vi "NMRFMswitch.vi"() -> ()   [LabVIEW 2018]
uses:
  <vilib>/Analysis/2dsp.llb/Power Spectrum (DBL).vi
  rssmt/RunNumberGlobal.vi
  kleinjan/MKS/Global - Pressure & Flow.vi
  <vilib>/Analysis/NI_AALBase.lvlib
  <vilib>/Analysis/NI_AALPro.lvlib
panel:
  in  "RunNumber":dbl format="%#_13g"
  out "Peak Amp":dbl(graph)=74.1337708971354
  out "Python OK":bool=TRUE
  out "Polarization":sgl=1.7080129 format="%.3f"
  out "+3.3V OK":bool=TRUE
  out "Qsub OK":bool
  out "standard error":string
  out "standard output":string
  out "return code":i32
  out "initphase":dbl=2.09 format="%#_13g"
  out "inittune":dbl=3.248 format="%#_13g"
  in  "Save Tune":bool
  in  "Tune?":bool=TRUE
  out "Date / Time":string="12/21/2021 3:07:32 PM"
  in  "Stop Run":bool=TRUE
  out "He readback":bool
  in  "Prompt?":bool
  out "He temp (K)":sgl=2.13326 format="%.3f"
  out "He press (torr)":sgl=33.89 format="%.3f"
  in  "NMR Channel Select":string(combo)="Tune1.csv"
  out "Color Box":u32(colorbox)=16711680
  out "Measurement":enum16{"TEQ", "POL", "QCV"}(ring)=enum."QCV"
  in  "VME IP Address":string="192.168.24.146"
  out "FFT Vrms":dbl[](graph)=[0.005219076637020729, 0.0039878980940110925, 0.0036329447037529434, 0.003167506199185892, 0.002848999314516927, 0.0024923420584089507, 0.002185783432691833, 0.0019623062753076612, 0.0017456237192042675, 0.0015310589705579407, 0.0013569206947159228, 0.0012134296553531008, 0.0010661913882126185, 0.0009417865401198701, 0.0008289553058562431, 0.0007426697969914733, 0.0006543871227562969, 0.0005691981056566225, 0.0004985796296117873, 0.000444582165316538, 0.0003908334146047696, 0.00034689887876954856, 0.00029774652842368897, 0.0002704403862780026, 0.0002271604793132453, 0.00020413555661144572, 0.00017624411940442264, 0.00015585149747815723, 0.00013132078167075022, 0.0001195156866464364, 0.00010987586628788737, 8.462443756275535e-05, 7.876977088235619e-05, 6.70471531529734e-05, 6.782696234467443e-05, 5.204485709629659e-05, 4.2881690215771905e-05, 2.868837131108542e-05, 3.646022540118467e-05, 2.5174670763212626e-05, 2.4275865918577663e-05, 1.977860163321803e-05, 2.0218195658450144e-05, 1.5094086218758437e-05, 1.0805592250755934e-05, 1.1612054327236393e-05, 1.0702829004656882e-05, 6.927920054257791e-06, 8.444237907182155e-06, 4.302452084273682e-06, 5.339321799968253e-06, 7.218121245343906e-06, 3.7765728081436e-06, 2.8602044585862934e-06, 4.859347329579347e-06, 5.065161881862085e-06, 2.3556171895703534e-06, 1.7632661431426266e-06, 3.379390145710016e-06, 2.7603757096228226e-06, 3.6214619183540137e-06, 3.3344073928151306e-06, 1.102179735422125e-06, 1.0412493305540784e-05, 2.523883779132704e-06, 5.9409226720671005e-06, 3.4619760167465126e-07, 9.010440109742317e-07, 2.401774338798568e-07, 5.3535552158452226e-06, 3.6940163929523105e-06, 3.4039009222603295e-06, 4.582524510322615e-06, 2.513437155372671e-06, 3.895119393056086e-06, 7.346211597269102e-06, 7.126116644995652e-06, 6.049774016482352e-06, 8.854330148411976e-06, 9.192536011516818e-07, 7.232552250072598e-06, 7.328129506360153e-06, 6.413204468246682e-06, 6.579066941521174e-06, 4.988346286272407e-06, 3.865009185428311e-06, 5.9602567586528205e-06, 6.379649198485404e-06, 1.9180240572629512e-06, 2.4865392439123074e-06, 4.077423508916666e-06, 2.6143194254198198e-06, 1.1582615724765671e-06, 2.8823995318867116e-06, 6.385725297552865e-06, 7.387976979956906e-06, 1.962928382011928e-06, 5.487268486039249e-06, 4.542898540052593e-06, 3.920885322308244e-06, 2.560006411681713e-06, 6.030758252294827e-06, 2.8147731643947036e-06, 3.767037305710274e-06, 2.2940292462848864e-06, 6.082474368564689e-07, 3.32627146099113e-06, 1.4201614366018455e-06, 2.990764004313556e-06, 5.798579609053757e-06, 8.551040913858013e-06, 6.487437175474049e-06, 5.280254351335599e-06, 3.2689120370825972e-06, 3.024531763084045e-06, 5.816131915181896e-06, 2.084880682526168e-06, 4.749183768250868e-06, 2.5155270391606587e-06, 5.161404132650414e-06, 8.948372740255112e-06, 3.7134069338070665e-06, 1.0504243435692216e-06, 2.486546756935266e-06, 5.708480201850752e-06, 3.4078826415869943e-06, 2.7526388449297627e-06, 8.105361535117322e-06, 1.4868612920884835e-06, 2.3496303492346643e-06, 3.1063386478581925e-06, 1.6041115487796047e-06, 2.5868779778952035e-06, 5.345577459310027e-06, 1.9006938798563804e-06, 4.397705633197135e-06, 3.38743005875455e-06, 1.4982947809591981e-06, 2.6902031437364864e-06, 3.732947753472797e-06, 2.3609284770920314e-06, 9.243175552374334e-06, 3.912353690878166e-06, 4.4078681623996285e-06, 3.838535836859122e-06, 3.3526472596387042e-06, 4.571851526932495e-06, 2.4329647044319065e-06, 2.497090370438281e-06, 4.215928959236651e-06, 4.9956874449258715e-06, 3.993018282604913e-06, 4.835554673477225e-06, 2.6850490929158865e-06, 4.737311136731914e-06, 1.9370086076116144e-06, 1.6342895919624075e-06, 1.5865940297551477e-06, 2.3464563158779775e-06, 3.8000988173413713e-06, 2.3042989349919555e-06, 4.252040733881927e-06, 5.922353590007147e-06, 4.960033169847504e-06, 8.415695746076422e-07, 2.5973560267739965e-06, 4.145285922687817e-06, 1.4972808238134822e-06, 3.6651950916562555e-06, 7.692102378806355e-06, 2.252172769669826e-06, 2.528448476027188e-06, 1.7270842871089151e-06, 8.732998643384956e-07, 1.941128023169817e-06, 4.967581144990737e-07, 2.122261572666148e-06, 2.7403051949501256e-06, 2.4487149582217077e-06, 4.695501688085451e-06, 4.028757067113805e-06, 3.994650398277535e-06, 1.321960383008639e-06, 7.229471979478003e-06, 2.8630109874025474e-06, 4.835926382490523e-06, 5.328936669165124e-06, 3.2295568028357553e-06, 4.122039456315995e-06, 4.415345749314911e-06, 2.0464868375281003e-06, 2.116876710242299e-06, 4.34647621603492e-06, 7.346635334484221e-06, 3.735213245442724e-06, 1.4876587271631782e-06, 2.3704959917761274e-06, 2.23938979663892e-06, 3.6731417379864763e-06, 2.541846286331768e-06, 1.6299280662148296e-06, 1.6299280662148296e-06, 2.541846286331768e-06, 3.6731417379864763e-06, 2.23938979663892e-06, 2.3704959917761274e-06, 1.4876587271631782e-06, 3.735213245442724e-06, 7.346635334484221e-06, 4.34647621603492e-06, 2.116876710242299e-06, 2.0464868375281003e-06, 4.415345749314911e-06, 4.122039456315995e-06, 3.2295568028357553e-06, 5.328936669165124e-06, 4.835926382490523e-06, 2.8630109874025474e-06, 7.229471979478003e-06, 1.321960383008639e-06, 3.994650398277535e-06, 4.028757067113805e-06, 4.695501688085451e-06, 2.4487149582217077e-06, 2.7403051949501256e-06, 2.122261572666148e-06, 4.967581144990737e-07, 1.941128023169817e-06, 8.732998643384956e-07, 1.7270842871089151e-06, 2.528448476027188e-06, 2.252172769669826e-06, 7.692102378806355e-06, 3.6651950916562555e-06, 1.4972808238134822e-06, 4.145285922687817e-06, 2.5973560267739965e-06, 8.415695746076422e-07, 4.960033169847504e-06, 5.922353590007147e-06, 4.252040733881927e-06, 2.3042989349919555e-06, 3.8000988173413713e-06, 2.3464563158779775e-06, 1.5865940297551477e-06, 1.6342895919624075e-06, 1.9370086076116144e-06, 4.737311136731914e-06, 2.6850490929158865e-06, 4.835554673477225e-06, 3.993018282604913e-06, 4.9956874449258715e-06, 4.215928959236651e-06, 2.497090370438281e-06, 2.4329647044319065e-06, 4.571851526932495e-06, 3.3526472596387042e-06, 3.838535836859122e-06, 4.4078681623996285e-06, 3.912353690878166e-06, 9.243175552374334e-06, 2.3609284770920314e-06, 3.732947753472797e-06, 2.6902031437364864e-06, 1.4982947809591981e-06, 3.38743005875455e-06, 4.397705633197135e-06, 1.9006938798563804e-06, 5.345577459310027e-06, 2.5868779778952035e-06, 1.6041115487796047e-06, 3.1063386478581925e-06, 2.3496303492346643e-06, 1.4868612920884835e-06, 8.105361535117322e-06, 2.7526388449297627e-06, 3.4078826415869943e-06, 5.708480201850752e-06, 2.486546756935266e-06, 1.0504243435692216e-06, 3.7134069338070665e-06, 8.948372740255112e-06, 5.161404132650414e-06, 2.5155270391606587e-06, 4.749183768250868e-06, 2.084880682526168e-06, 5.816131915181896e-06, 3.024531763084045e-06, 3.2689120370825972e-06, 5.280254351335599e-06, 6.487437175474049e-06, 8.551040913858013e-06, 5.798579609053757e-06, 2.990764004313556e-06, 1.4201614366018455e-06, 3.32627146099113e-06, 6.082474368564689e-07, 2.2940292462848864e-06, 3.767037305710274e-06, 2.8147731643947036e-06, 6.030758252294827e-06, 2.560006411681713e-06, 3.920885322308244e-06, 4.542898540052593e-06, 5.487268486039249e-06, 1.962928382011928e-06, 7.387976979956906e-06, 6.385725297552865e-06, 2.8823995318867116e-06, 1.1582615724765671e-06, 2.6143194254198198e-06, 4.077423508916666e-06, 2.4865392439123074e-06, 1.9180240572629512e-06, 6.379649198485404e-06, 5.9602567586528205e-06, 3.865009185428311e-06, 4.988346286272407e-06, 6.579066941521174e-06, 6.413204468246682e-06, 7.328129506360153e-06, 7.232552250072598e-06, 9.192536011516818e-07, 8.854330148411976e-06, 6.049774016482352e-06, 7.126116644995652e-06, 7.346211597269102e-06, 3.895119393056086e-06, 2.513437155372671e-06, 4.582524510322615e-06, 3.4039009222603295e-06, 3.6940163929523105e-06, 5.3535552158452226e-06, 2.401774338798568e-07, 9.010440109742317e-07, 3.4619760167465126e-07, 5.9409226720671005e-06, 2.523883779132704e-06, 1.0412493305540784e-05, 1.102179735422125e-06, 3.3344073928151306e-06, 3.6214619183540137e-06, 2.7603757096228226e-06, 3.379390145710016e-06, 1.7632661431426266e-06, 2.3556171895703534e-06, 5.065161881862085e-06, 4.859347329579347e-06, 2.8602044585862934e-06, 3.7765728081436e-06, 7.218121245343906e-06, 5.339321799968253e-06, 4.302452084273682e-06, 8.444237907182155e-06, 6.927920054257791e-06, 1.0702829004656882e-05, 1.1612054327236393e-05, 1.0805592250755934e-05, 1.5094086218758437e-05, 2.0218195658450144e-05, 1.977860163321803e-05, 2.4275865918577663e-05, 2.5174670763212626e-05, 3.646022540118467e-05, 2.868837131108542e-05, 4.2881690215771905e-05, 5.204485709629659e-05, 6.782696234467443e-05, 6.70471531529734e-05, 7.876977088235619e-05, 8.462443756275535e-05, 0.00010987586628788737, 0.0001195156866464364, 0.00013132078167075022, 0.00015585149747815723, 0.00017624411940442264, 0.00020413555661144572, 0.0002271604793132453, 0.0002704403862780026, 0.00029774652842368897, 0.00034689887876954856, 0.0003908334146047696, 0.000444582165316538, 0.0004985796296117873, 0.0005691981056566225, 0.0006543871227562969, 0.0007426697969914733, 0.0008289553058562431, 0.0009417865401198701, 0.0010661913882126185, 0.0012134296553531008, 0.0013569206947159228, 0.0015310589705579407, 0.0017456237192042675, 0.0019623062753076612, 0.002185783432691833, 0.0024923420584089507, 0.002848999314516927, 0.003167506199185892, 0.0036329447037529434, 0.0039878980940110925]
  out "Raw NMR Graph / Ave":cluster{dbl, "Step Width (MHz)":dbl, dbl[][]}(graph)={224.25, "Step Width (MHz)"=0.001, [[0.0013885498046875, 0.001312255859375, 0.0015411376953125, 0.0014190673828125, 0.00146484375, 0.0015106201171875, 0.00146484375, 0.0014801025390625, 0.001434326171875, 0.001373291015625, 0.0012969970703125, 0.0012969970703125, 0.0012969970703125, 0.00140380859375, 0.001373291015625, 0.0013275146484375, 0.001373291015625, 0.0013885498046875, 0.001373291015625, 0.0013427734375, 0.0013580322265625, 0.001495361328125, 0.0012969970703125, 0.0011138916015625, 0.0013885498046875, 0.001251220703125, 0.0012969970703125, 0.001220703125, 0.001220703125, 0.0013275146484375, 0.00140380859375, 0.00140380859375, 0.00146484375, 0.0013427734375, 0.0012359619140625, 0.00140380859375, 0.0012664794921875, 0.001312255859375, 0.0013427734375, 0.00128173828125, 0.001129150390625, 0.0012359619140625, 0.0012664794921875, 0.0012054443359375, 0.0012054443359375, 0.0012664794921875, 0.0012359619140625, 0.001220703125, 0.001129150390625, 0.000946044921875, 0.0012359619140625, 0.0010833740234375, 0.0010986328125, 0.001068115234375, 0.0012054443359375, 0.00115966796875, 0.0012359619140625, 0.00115966796875, 0.0010223388671875, 0.001068115234375, 0.001220703125, 0.0011138916015625, 0.00103759765625, 0.0010833740234375, 0.0010528564453125, 0.0009307861328125, 0.000946044921875, 0.001068115234375, 0.001190185546875, 0.00115966796875, 0.001190185546875, 0.0012969970703125, 0.0012664794921875, 0.0010528564453125, 0.001129150390625, 0.001312255859375, 0.001190185546875, 0.0011138916015625, 0.001129150390625, 0.0011444091796875, 0.0011749267578125, 0.0012359619140625, 0.0010833740234375, 0.001190185546875, 0.0010833740234375, 0.0011444091796875, 0.001129150390625, 0.001190185546875, 0.0013580322265625, 0.0013275146484375, 0.0012969970703125, 0.00128173828125, 0.001251220703125, 0.00115966796875, 0.001220703125, 0.0013580322265625, 0.0012969970703125, 0.0012664794921875, 0.0013885498046875, 0.0013580322265625, 0.001434326171875, 0.0015106201171875, 0.0014190673828125, 0.001312255859375, 0.0015411376953125, 0.0013580322265625, 0.001190185546875, 0.001556396484375, 0.001495361328125, 0.001495361328125, 0.0015869140625, 0.0015869140625, 0.00152587890625, 0.0016937255859375, 0.001708984375, 0.0017852783203125, 0.001556396484375, 0.00152587890625, 0.0017852783203125, 0.0016326904296875, 0.0016937255859375, 0.00177001953125, 0.00177001953125, 0.0018463134765625, 0.00189208984375, 0.0018463134765625, 0.0019073486328125, 0.0017852783203125, 0.0019378662109375, 0.001922607421875, 0.002044677734375, 0.00201416015625, 0.001983642578125, 0.002044677734375, 0.0020751953125, 0.0022735595703125, 0.002227783203125, 0.0022430419921875, 0.0023345947265625, 0.00244140625, 0.002471923828125, 0.0027008056640625, 0.0025787353515625, 0.002685546875, 0.0028228759765625, 0.0028839111328125, 0.0029296875, 0.003143310546875, 0.003143310546875, 0.0031585693359375, 0.0032501220703125, 0.0034637451171875, 0.003570556640625, 0.0037078857421875, 0.00390625, 0.0040740966796875, 0.0041351318359375, 0.0042572021484375, 0.0045013427734375, 0.0045623779296875, 0.0048675537109375, 0.0052032470703125, 0.00543212890625, 0.005645751953125, 0.0059967041015625, 0.006378173828125, 0.00665283203125, 0.0069732666015625, 0.00738525390625, 0.007904052734375, 0.0084228515625, 0.0091400146484375, 0.009552001953125, 0.0103302001953125, 0.0110015869140625, 0.0119171142578125, 0.0129852294921875, 0.0140533447265625, 0.0154876708984375, 0.016815185546875, 0.0185546875, 0.02069091796875, 0.0230865478515625, 0.0256195068359375, 0.02874755859375, 0.0323333740234375, 0.0367584228515625, 0.0414581298828125, 0.046661376953125, 0.0526123046875, 0.058868408203125, 0.0647125244140625, 0.06964111328125, 0.0731658935546875, 0.074798583984375, 0.0745697021484375, 0.0721588134765625, 0.0679473876953125, 0.062469482421875, 0.05633544921875, 0.0499114990234375, 0.044036865234375, 0.0384979248046875, 0.033599853515625, 0.0293121337890625, 0.025787353515625, 0.02276611328125, 0.0201416015625, 0.017913818359375, 0.0159759521484375, 0.0142974853515625, 0.0130767822265625, 0.0119171142578125, 0.0106658935546875, 0.0097808837890625, 0.00909423828125, 0.00830078125, 0.00762939453125, 0.00714111328125, 0.0065765380859375, 0.006256103515625, 0.0059051513671875, 0.005462646484375, 0.005126953125, 0.004852294921875, 0.0044097900390625, 0.0040435791015625, 0.0039520263671875, 0.004150390625, 0.0038604736328125, 0.0036163330078125, 0.0033416748046875, 0.0032806396484375, 0.0029449462890625, 0.0030975341796875, 0.002716064453125, 0.002532958984375, 0.00244140625, 0.002532958984375, 0.0022430419921875, 0.002349853515625, 0.0022430419921875, 0.00213623046875, 0.0021514892578125, 0.0018463134765625, 0.001983642578125, 0.0017852783203125, 0.00177001953125, 0.0017852783203125, 0.0018157958984375, 0.0015869140625, 0.00164794921875, 0.001617431640625, 0.0017242431640625, 0.0016021728515625, 0.0014495849609375, 0.0013427734375, 0.0012969970703125, 0.00140380859375, 0.0011749267578125, 0.0012969970703125, 0.0012359619140625, 0.0011138916015625, 0.001190185546875, 0.0011138916015625, 0.0013427734375, 0.001190185546875, 0.00115966796875, 0.0010986328125, 0.0010833740234375, 0.001068115234375, 0.0010833740234375, 0.00115966796875, 0.0010528564453125, 0.001190185546875, 0.0011749267578125, 0.001068115234375, 0.000946044921875, 0.0009613037109375, 0.0009765625, 0.0012054443359375, 0.000885009765625, 0.0010986328125, 0.0009613037109375, 0.0008697509765625, 0.001068115234375, 0.0010223388671875, 0.001129150390625, 0.0010528564453125, 0.0012359619140625, 0.0012359619140625, 0.001129150390625, 0.0012664794921875, 0.00115966796875, 0.0012664794921875, 0.001068115234375, 0.0012054443359375, 0.0014190673828125, 0.001434326171875, 0.001312255859375, 0.001312255859375, 0.00115966796875, 0.0012359619140625, 0.0013580322265625, 0.00115966796875, 0.001190185546875, 0.0010223388671875, 0.000946044921875, 0.00103759765625, 0.0010833740234375, 0.0008392333984375, 0.0009307861328125, 0.0008392333984375, 0.0009765625, 0.000823974609375, 0.0008087158203125, 0.0007171630859375, 0.0007781982421875, 0.0007476806640625, 0.0008544921875, 0.0006256103515625, 0.0007476806640625, 0.00091552734375, 0.000762939453125, 0.0006866455078125, 0.0008544921875, 0.00067138671875, 0.0007476806640625, 0.000732421875, 0.00067138671875, 0.000762939453125, 0.0007476806640625, 0.0008087158203125, 0.0006866455078125, 0.000640869140625, 0.0005950927734375, 0.000640869140625, 0.000946044921875, 0.00067138671875, 0.0007476806640625, 0.00079345703125, 0.0009002685546875, 0.0008544921875, 0.00067138671875, 0.00079345703125, 0.0008087158203125, 0.000885009765625, 0.000823974609375, 0.0007476806640625, 0.0008087158203125, 0.0008697509765625, 0.000823974609375, 0.0008392333984375, 0.0009307861328125, 0.0007781982421875, 0.000732421875, 0.000762939453125, 0.0008697509765625, 0.0006866455078125, 0.0006256103515625, 0.000823974609375, 0.0009307861328125, 0.0008392333984375, 0.001068115234375, 0.0008087158203125, 0.0008087158203125, 0.0009307861328125, 0.001068115234375, 0.000946044921875, 0.0009002685546875, 0.0008697509765625, 0.001129150390625, 0.0010986328125, 0.00091552734375, 0.001068115234375, 0.0009002685546875, 0.00091552734375, 0.0009765625, 0.0009613037109375, 0.000823974609375, 0.0008087158203125, 0.00103759765625, 0.0012969970703125, 0.0009918212890625, 0.00103759765625, 0.0010528564453125, 0.0011138916015625, 0.000946044921875, 0.0010528564453125, 0.0010528564453125, 0.00091552734375, 0.0010833740234375, 0.0010986328125, 0.00115966796875, 0.001190185546875, 0.001220703125, 0.001251220703125, 0.0011138916015625, 0.0012359619140625, 0.0012359619140625, 0.001312255859375], [0.0, 0.0, 0.0, 0.0, 0.0, 0.0, 0.0, 0.0, 0.0, 0.0, 0.0, 0.0, 0.0, 0.0, 0.0, 0.0, 0.0, 0.0, 0.0, 0.0, 0.0, 0.0, 0.0, 0.0, 0.0, 0.0, 0.0, 0.0, 0.0, 0.0, 0.0, 0.0, 0.0, 0.0, 0.0, 0.0, 0.0, 0.0, 0.0, 0.0, 0.0, 0.0, 0.0, 0.0, 0.0, 0.0, 0.0, 0.0, 0.0, 0.0, 0.0, 0.0, 0.0, 0.0, 0.0, 0.0, 0.0, 0.0, 0.0, 0.0, 0.0, 0.0, 0.0, 0.0, 0.0, 0.0, 0.0, 0.0, 0.0, 0.0, 0.0, 0.0, 0.0, 0.0, 0.0, 0.0, 0.0, 0.0, 0.0, 0.0, 0.0, 0.0, 0.0, 0.0, 0.0, 0.0, 0.0, 0.0, 0.0, 0.0, 0.0, 0.0, 0.0, 0.0, 0.0, 0.0, 0.0, 0.0, 0.0, 0.0, 0.0, 0.0, 0.0, 0.0, 0.0, 0.0, 0.0, 0.0, 0.0, 0.0, 0.0, 0.0, 0.0, 0.0, 0.0, 0.0, 0.0, 0.0, 0.0, 0.0, 0.0, 0.0, 0.0, 0.0, 0.0, 0.0, 0.0, 0.0, 0.0, 0.0, 0.0, 0.0, 0.0, 0.0, 0.0, 0.0, 0.0, 0.0, 0.0, 0.0, 0.0, 0.0, 0.0, 0.0, 0.0, 0.0, 0.0, 0.0, 0.0, 0.0, 0.0, 0.0, 0.0, 0.0, 0.0, 0.0, 0.0, 0.0, 0.0, 0.0, 0.0, 0.0, 0.0, 0.0, 0.0, 0.0, 0.0, 0.0, 0.0, 0.0, 0.0, 0.0, 0.0, 0.0, 0.0, 0.0, 0.0, 0.0, 0.0, 0.0, 0.0, 0.0, 0.0, 0.0, 0.0, 0.0, 0.0, 0.0, 0.0, 0.0, 0.0, 0.0, 0.0, 0.0, 0.0, 0.0, 0.0, 0.0, 0.0, 0.0, 0.0, 0.0, 0.0, 0.0, 0.0, 0.0, 0.0, 0.0, 0.0, 0.0, 0.0, 0.0, 0.0, 0.0, 0.0, 0.0, 0.0, 0.0, 0.0, 0.0, 0.0, 0.0, 0.0, 0.0, 0.0, 0.0, 0.0, 0.0, 0.0, 0.0, 0.0, 0.0, 0.0, 0.0, 0.0, 0.0, 0.0, 0.0, 0.0, 0.0, 0.0, 0.0, 0.0, 0.0, 0.0, 0.0, 0.0, 0.0, 0.0, 0.0, 0.0, 0.0, 0.0, 0.0, 0.0, 0.0, 0.0, 0.0, 0.0, 0.0, 0.0, 0.0, 0.0, 0.0, 0.0, 0.0, 0.0, 0.0, 0.0, 0.0, 0.0, 0.0, 0.0, 0.0, 0.0, 0.0, 0.0, 0.0, 0.0, 0.0, 0.0, 0.0, 0.0, 0.0, 0.0, 0.0, 0.0, 0.0, 0.0, 0.0, 0.0, 0.0, 0.0, 0.0, 0.0, 0.0, 0.0, 0.0, 0.0, 0.0, 0.0, 0.0, 0.0, 0.0, 0.0, 0.0, 0.0, 0.0, 0.0, 0.0, 0.0, 0.0, 0.0, 0.0, 0.0, 0.0, 0.0, 0.0, 0.0, 0.0, 0.0, 0.0, 0.0, 0.0, 0.0, 0.0, 0.0, 0.0, 0.0, 0.0, 0.0, 0.0, 0.0, 0.0, 0.0, 0.0, 0.0, 0.0, 0.0, 0.0, 0.0, 0.0, 0.0, 0.0, 0.0, 0.0, 0.0, 0.0, 0.0, 0.0, 0.0, 0.0, 0.0, 0.0, 0.0, 0.0, 0.0, 0.0, 0.0, 0.0, 0.0, 0.0, 0.0, 0.0, 0.0, 0.0, 0.0, 0.0, 0.0, 0.0, 0.0, 0.0, 0.0, 0.0, 0.0, 0.0, 0.0, 0.0, 0.0, 0.0, 0.0, 0.0, 0.0, 0.0, 0.0, 0.0, 0.0, 0.0, 0.0, 0.0, 0.0, 0.0, 0.0, 0.0, 0.0, 0.0, 0.0, 0.0, 0.0, 0.0, 0.0], [0.000884405500000046, 0.000875605500000004, 0.0008668494999999623, 0.0008581375000001678, 0.0008494695000001258, 0.000840845500000084, 0.0008322655000000428, 0.0008237295000000018, 0.0008152374999999615, 0.0008067895000001609, 0.00079838550000012, 0.0007900255000000796, 0.0007817095000000395, 0.0007734374999999999, 0.0007652094999999607, 0.0007570255000001541, 0.0007488855000001145, 0.0007407895000000752, 0.0007327375000000365, 0.0007247294999999981, 0.0007167654999999602, 0.0007088455000001472, 0.0007009695000001089, 0.0006931375000000709, 0.0006853495000000335, 0.0006776054999999964, 0.0006699054999999598, 0.0006622495000001405, 0.0006546375000001035, 0.0006470695000000669, 0.0006395455000000307, 0.0006320654999999949, 0.0006246294999999595, 0.000617237500000134, 0.0006098895000000983, 0.0006025855000000629, 0.0005953255000000279, 0.0005881094999999934, 0.0005809374999999593, 0.0005738095000001277, 0.0005667255000000931, 0.000559685500000059, 0.0005526895000000253, 0.0005457374999999921, 0.0005388294999999593, 0.0005319655000001213, 0.0005251455000000881, 0.0005183695000000552, 0.0005116375000000228, 0.0005049494999999909, 0.0004983054999999593, 0.0004917055000001151, 0.00048514950000008315, 0.0004786375000000516, 0.0004721695000000205, 0.00046574549999998976, 0.0004593654999999595, 0.0004530295000001091, 0.0004467375000000784, 0.0004404895000000481, 0.00043428550000001824, 0.0004281254999999888, 0.0004220094999999598, 0.0004159375000001032, 0.0004099095000000737, 0.00040392550000004475, 0.0003979855000000161, 0.00039208949999998795, 0.0003862374999999602, 0.0003804295000000973, 0.0003746655000000691, 0.00036894550000004145, 0.00036326950000001415, 0.0003576374999999872, 0.0003520494999999607, 0.00034650550000009167, 0.00034100550000006475, 0.0003355495000000383, 0.00033013750000001225, 0.0003247694999999866, 0.0003194454999999614, 0.0003141655000000861, 0.00030892950000006045, 0.00030373750000003524, 0.00029858950000001045, 0.00029348549999998614, 0.00028842549999996215, 0.0002834095000000806, 0.00027843750000005626, 0.00027350950000003233, 0.00026862550000000883, 0.00026378549999998575, 0.0002589894999999631, 0.00025423750000007524, 0.0002495295000000522, 0.00024486550000002953, 0.00024024550000000731, 0.00023566949999998546, 0.00023113749999996411, 0.00022664950000007007, 0.00022220550000004826, 0.00021780550000002687, 0.00021344950000000589, 0.00020913749999998534, 0.00020486949999996525, 0.00020064550000006495, 0.00019646550000004443, 0.0001923295000000243, 0.0001882375000000046, 0.00018418949999998537, 0.00018018549999996648, 0.00017622550000005998, 0.0001723095000000407, 0.00016843750000002187, 0.00016460950000000345, 0.00016082549999998544, 0.00015708549999996787, 0.00015338950000005512, 0.00014973750000003713, 0.00014612950000001957, 0.0001425655000000024, 0.00013904549999998566, 0.00013556949999996937, 0.0001321375000000504, 0.00012874950000003367, 0.00012540550000001736, 0.00012210550000000148, 0.00011884949999998602, 0.00011563750000006164, 0.00011246950000004579, 0.00010934550000003033, 0.00010626550000001528, 0.00010322950000000068, 0.00010023749999998649, 9.728950000005588e-05, 9.438550000004129e-05, 9.152550000002709e-05, 8.870950000001334e-05, 8.59375e-05, 8.320949999998707e-05, 8.052550000005024e-05, 7.78855000000369e-05, 7.528950000002399e-05, 7.273750000001149e-05, 7.022949999999943e-05, 6.776549999998778e-05, 6.534550000004471e-05, 6.296950000003266e-05, 6.0637500000021e-05, 5.8349500000009786e-05, 5.6105499999998984e-05, 5.390549999998861e-05, 5.17495000000393e-05, 4.963750000002851e-05, 4.756950000001814e-05, 4.554550000000819e-05, 4.356549999999866e-05, 4.162949999998955e-05, 3.9737500000034014e-05, 3.788950000002449e-05, 3.6085500000015394e-05, 3.432550000000672e-05, 3.260949999999846e-05, 3.093749999999062e-05, 2.9309500000028848e-05, 2.77255000000206e-05, 2.618550000001277e-05, 2.468950000000536e-05, 2.3237499999998376e-05, 2.1829499999991806e-05, 2.0465500000023797e-05, 1.914550000001682e-05, 1.7869500000010265e-05, 1.6637500000004125e-05, 1.5449499999998406e-05, 1.430549999999311e-05, 1.3205500000018873e-05, 1.2149500000013166e-05, 1.1137500000007877e-05, 1.016950000000301e-05, 9.245499999998563e-06, 8.365499999994538e-06, 7.5295000000140655e-06, 6.7375000000096285e-06, 5.989500000005612e-06, 5.2855000000020156e-06, 4.625499999998839e-06, 4.009499999996083e-06, 3.4375000000093793e-06, 2.9095000000062124e-06, 2.4255000000034664e-06, 1.9855000000011404e-06, 1.5894999999992347e-06, 1.237499999997749e-06, 9.295000000048122e-07, 6.655000000029163e-07, 4.455000000014406e-07, 2.6950000000038516e-07, 1.374999999997499e-07, 4.9499999999534794e-08, 5.500000000365162e-09, 5.499999999739884e-09, 4.9499999999534794e-08, 1.374999999997499e-07, 2.6950000000038516e-07, 4.455000000014406e-07, 6.654999999960382e-07, 9.294999999966835e-07, 1.237499999997749e-06, 1.5894999999992347e-06, 1.9855000000011404e-06, 2.4255000000034664e-06, 2.9094999999918315e-06, 3.437499999993747e-06, 4.009499999996083e-06, 4.625499999998839e-06, 5.2855000000020156e-06, 5.989500000005612e-06, 6.737499999987744e-06, 7.5294999999909305e-06, 8.365499999994538e-06, 9.245499999998563e-06, 1.016950000000301e-05, 1.1137500000007877e-05, 1.2149499999983777e-05, 1.3205499999988236e-05, 1.430549999999311e-05, 1.5449499999998406e-05, 1.6637500000004125e-05, 1.7869500000010265e-05, 1.914549999997993e-05, 2.0465499999985657e-05, 2.1829499999991806e-05, 2.3237499999998376e-05, 2.468950000000536e-05, 2.618550000001277e-05, 2.7725499999976206e-05, 2.93094999999832e-05, 3.093749999999062e-05, 3.260949999999846e-05, 3.432550000000672e-05, 3.6085500000015394e-05, 3.7889499999972594e-05, 3.973749999998087e-05, 4.162949999998955e-05, 4.356549999999866e-05, 4.554550000000819e-05, 4.756950000001814e-05, 4.9637499999969114e-05, 5.174949999997865e-05, 5.390549999998861e-05, 5.6105499999998984e-05, 5.8349500000009786e-05, 6.0637499999955355e-05, 6.296949999996573e-05, 6.534549999997655e-05, 6.776549999998778e-05, 7.022949999999943e-05, 7.273750000001149e-05, 7.528949999995083e-05, 7.788549999996248e-05, 8.052549999997458e-05, 8.320949999998707e-05, 8.59375e-05, 8.870950000001334e-05, 9.152549999994642e-05, 9.438549999995936e-05, 9.728949999997272e-05, 0.00010023749999998649, 0.00010322950000000068, 0.00010626550000001528, 0.00010934549999994216, 0.00011246949999995637, 0.00011563749999997098, 0.00011884949999998602, 0.00012210550000000148, 0.00012540550000001736, 0.000128749499999938, 0.00013213749999995347, 0.00013556949999996937, 0.00013904549999998566, 0.0001425655000000024, 0.00014612950000001957, 0.00014973749999993397, 0.0001533894999999507, 0.00015708549999996787, 0.00016082549999998544, 0.00016460950000000345, 0.00016843750000002187, 0.00017230949999993004, 0.00017622549999994806, 0.00018018549999996648, 0.00018418949999998537, 0.0001882375000000046, 0.0001923295000000243, 0.00019646549999992622, 0.00020064549999994553, 0.00020486949999996525, 0.00020913749999998534, 0.00021344950000000589, 0.00021780550000002687, 0.00022220549999992255, 0.00022664949999994313, 0.00023113749999996411, 0.00023566949999998546, 0.00024024550000000731, 0.00024486550000002953, 0.000249529499999919, 0.00025423749999994085, 0.0002589894999999631, 0.00026378549999998575, 0.00026862550000000883, 0.00027350950000003233, 0.0002784374999999156, 0.0002834094999999387, 0.00028842549999996215, 0.00029348549999998614, 0.00029858950000001045, 0.00030373750000003524, 0.00030892949999991224, 0.0003141654999999366, 0.0003194454999999614, 0.0003247694999999866, 0.00033013750000001225, 0.0003355495000000383, 0.00034100549999990906, 0.00034650549999993473, 0.0003520494999999607, 0.0003576374999999872, 0.00036326950000001415, 0.00036894550000004145, 0.00037466549999990594, 0.00038042949999993284, 0.0003862374999999602, 0.00039208949999998795, 0.0003979855000000161, 0.00040392550000004475, 0.00040990949999990305, 0.0004159374999999312, 0.0004220094999999598, 0.0004281254999999888, 0.00043428550000001824, 0.0004404895000000481, 0.00044673749999990016, 0.00045302949999992967, 0.0004593654999999595, 0.00046574549999998976, 0.0004721695000000205, 0.0004786375000000516, 0.00048514949999989743, 0.0004917054999999282, 0.0004983054999999593, 0.0005049494999999909, 0.0005116375000000228, 0.0005183695000000552, 0.0005251454999998949, 0.0005319654999999269, 0.0005388294999999593, 0.0005457374999999921, 0.0005526895000000253, 0.000559685500000059, 0.0005667254999998924, 0.0005738094999999257, 0.0005809374999999593, 0.0005881094999999934, 0.0005953255000000279, 0.0006025855000000629, 0.0006098894999998901, 0.0006172374999999246, 0.0006246294999999595, 0.0006320654999999949, 0.0006395455000000307, 0.0006470695000000669, 0.0006546374999998878, 0.0006622494999999236, 0.0006699054999999598, 0.0006776054999999964, 0.0006853495000000335, 0.000693137499999849, 0.0007009694999998856, 0.0007088454999999227, 0.0007167654999999602, 0.0007247294999999981, 0.0007327375000000365, 0.0007407894999998458, 0.0007488854999998836, 0.000757025499999922, 0.0007652094999999607, 0.0007734374999999999, 0.0007817095000000395, 0.0007900254999998427, 0.0007983854999998819, 0.0008067894999999214, 0.0008152374999999615, 0.0008237295000000018, 0.0008322655000000428, 0.0008408454999998396, 0.00084946949999988, 0.0008581374999999208, 0.0008668494999999623, 0.000875605500000004]]}
  in  "R&S GPIB Addr (28)":refnum<visa-resource-name>="GPIB0::28::INSTR"
  out "Pedestal (V)":dbl=0.0006638835872395818 format="%_2g"
  in  "Open Global Panel":bool=TRUE
  out "Peak center (MHz)":sgl=224.44414 format="%.3f"
  out "Telnet error out":errorcluster
  out "+3.3V supply":dbl=3.284 format="%_4g"
  out "Temp (C)":dbl=31.12 format="%_4g"
  out "RF level OK":bool=TRUE
  out "Polarization %":sgl=1.7080129 format="%.3e"
  out "# Good Spectra":i32=500
  out "Pedestal volts OK":bool=TRUE
  out "Sweep #":i32=6
  out "1st Sweep":bool
  out "ADC volts OK":bool=TRUE
  out "Peak Height Distribution":cluster{"Y":dbl[], "Y":dbl[]}[](graph)=[{"Y"=[1.68515093263186, 1.685512718520532, 1.6858745044092038, 1.6862362902978758, 1.6865980761865478, 1.6869598620752195, 1.6873216479638915, 1.6876834338525633, 1.6880452197412352, 1.688407005629907, 1.688768791518579, 1.6891305774072507, 1.6894923632959227, 1.6898541491845946, 1.6902159350732664, 1.6905777209619384, 1.6909395068506101, 1.691301292739282, 1.6916630786279538, 1.6920248645166258, 1.6923866504052976, 1.6927484362939695, 1.6931102221826415, 1.6934720080713133, 1.6938337939599852, 1.694195579848657, 1.694557365737329, 1.6949191516260007, 1.6952809375146727, 1.6956427234033447, 1.6960045092920164, 1.6963662951806884, 1.6967280810693601, 1.697089866958032, 1.6974516528467039, 1.6978134387353758, 1.6981752246240476, 1.6985370105127195, 1.6988987964013915, 1.6992605822900633, 1.6996223681787352, 1.699984154067407, 1.700345939956079, 1.7007077258447507, 1.7010695117334227, 1.7014312976220944, 1.7017930835107664, 1.7021548693994384, 1.7025166552881101, 1.702878441176782, 1.7032402270654539, 1.7036020129541258, 1.7039637988427976, 1.7043255847314696, 1.7046873706201415, 1.7050491565088133, 1.7054109423974853, 1.705772728286157, 1.706134514174829, 1.7064963000635007, 1.7068580859521727, 1.7072198718408444, 1.7075816577295164, 1.7079434436181884, 1.7083052295068601, 1.7086670153955321, 1.7090288012842039, 1.7093905871728758, 1.7097523730615476, 1.7101141589502196, 1.7104759448388913, 1.7108377307275633, 1.7111995166162353, 1.711561302504907, 1.711923088393579, 1.7122848742822507, 1.7126466601709227, 1.7130084460595945, 1.7133702319482664, 1.7137320178369384, 1.7140938037256102, 1.7144555896142821, 1.7148173755029539, 1.7151791613916259, 1.7155409472802976, 1.7159027331689696, 1.7162645190576413, 1.7166263049463133, 1.7169880908349853, 1.717349876723657, 1.717711662612329, 1.7180734485010007, 1.7184352343896727, 1.7187970202783445, 1.7191588061670164, 1.7195205920556882, 1.7198823779443602, 1.7202441638330321, 1.7206059497217039, 1.7209677356103759], "Y"=[1.0, 0.0, 1.0, 0.0, 2.0, 2.0, 2.0, 2.0, 0.0, 1.0, 1.0, 2.0, 2.0, 1.0, 0.0, 1.0, 1.0, 5.0, 0.0, 2.0, 1.0, 3.0, 1.0, 4.0, 3.0, 6.0, 3.0, 5.0, 2.0, 6.0, 8.0, 7.0, 8.0, 12.0, 12.0, 10.0, 9.0, 15.0, 3.0, 8.0, 11.0, 11.0, 9.0, 14.0, 14.0, 17.0, 9.0, 15.0, 13.0, 15.0, 9.0, 11.0, 9.0, 16.0, 7.0, 11.0, 9.0, 6.0, 8.0, 9.0, 8.0, 14.0, 8.0, 6.0, 8.0, 5.0, 6.0, 4.0, 5.0, 11.0, 4.0, 4.0, 1.0, 3.0, 5.0, 5.0, 5.0, 4.0, 2.0, 5.0, 1.0, 0.0, 1.0, 4.0, 1.0, 1.0, 1.0, 0.0, 0.0, 0.0, 1.0, 0.0, 0.0, 0.0, 0.0, 0.0, 1.0, 0.0, 0.0, 1.0]}]
  out "S/N":dbl=276.4068357498407 format="%_3g"
  out "Polarization %":dbl=1.7024247821191647 format="%_4g"
  out "Pedestal Diff (V)":sgl=-0.00033790368 format="%.4f"
  out "Peak amp (mV)":sgl=74.13377 format="%.4f"
  out "SMT error out":errorcluster
  out "Pol sdev":dbl=0.006159126917034453 format="%.3f"
  # "E1039 NMR Panel"
  # "Results"
  # "A\nv\ne\nr\na\ng\ne\ns"
  # "S\nw\ne\ne\np"
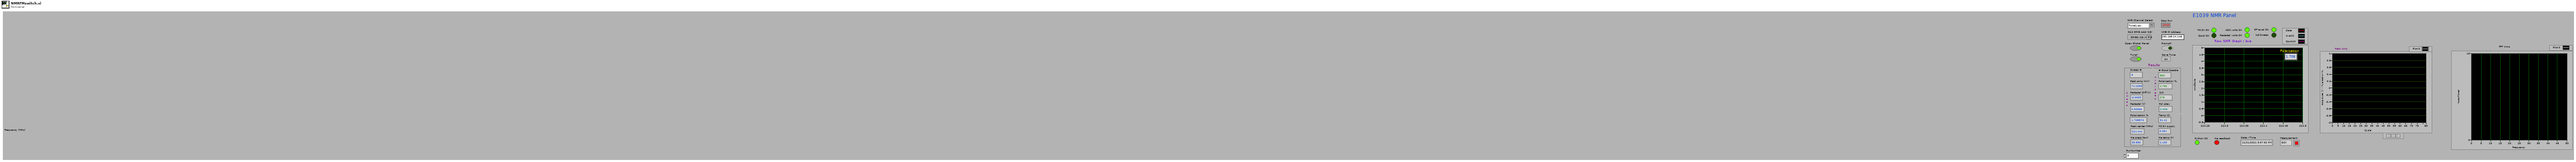
[diagram p1: front panel]
types:
  T1 = enum32{"Invalid", "Standard", "Closed", "Hidden", "Minimized", "Maximized"}
  T2 = enum32{"Bad", "Idle", "Run top level", "Running"}
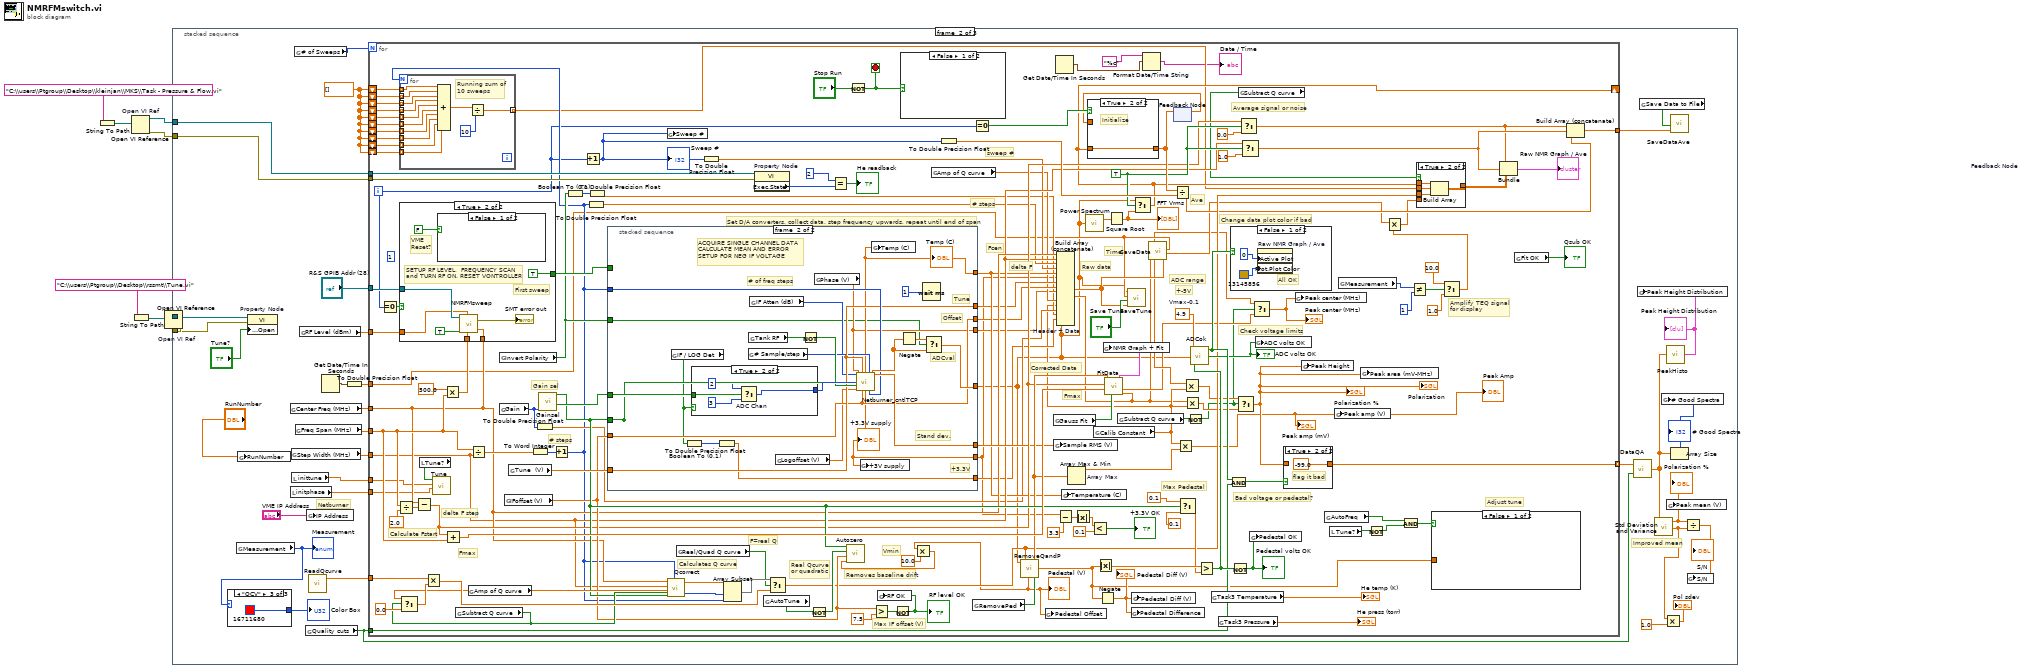
[diagram p0: block diagram]
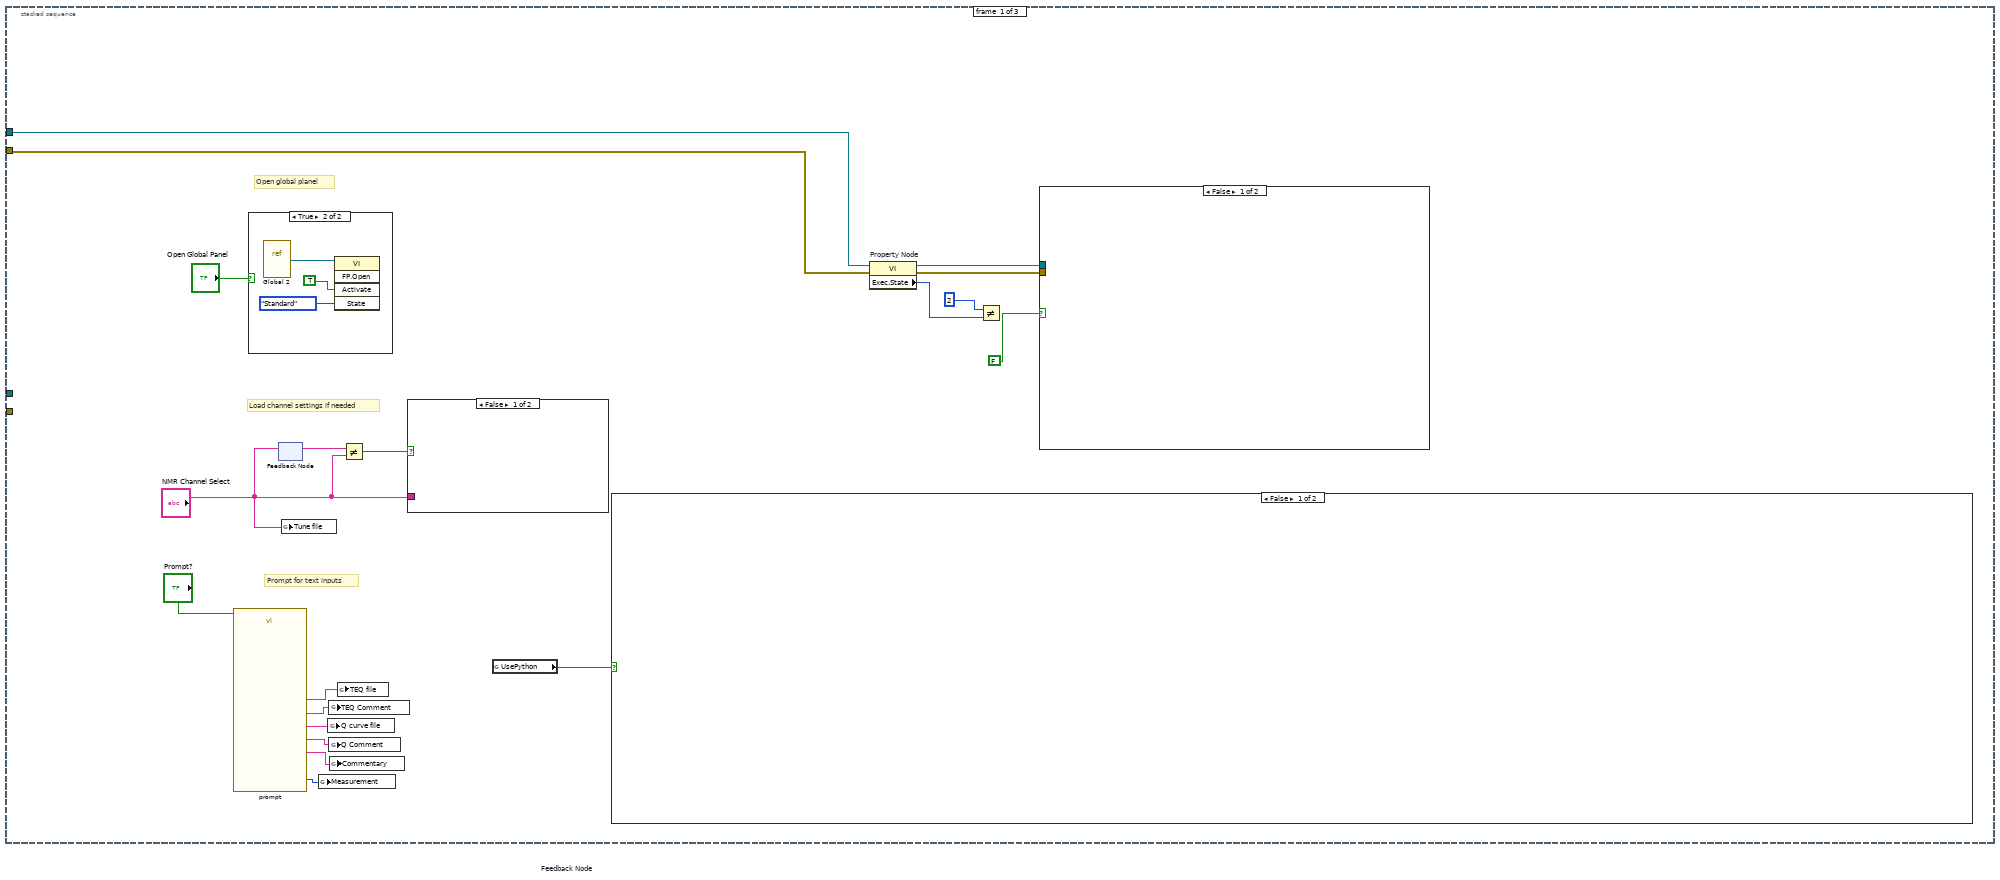
[diagram p2: hidden frame]
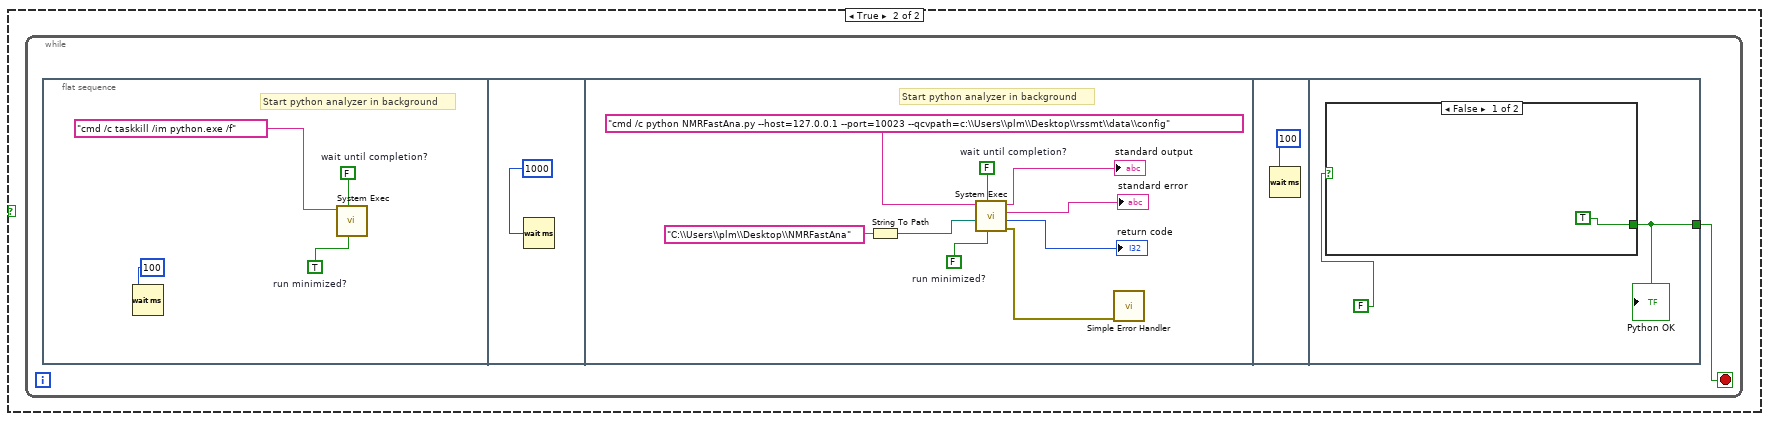
[diagram p3: hidden frame]
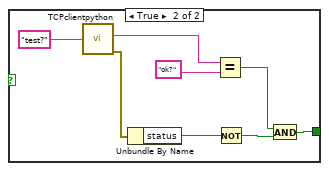
[diagram p4: hidden frame]
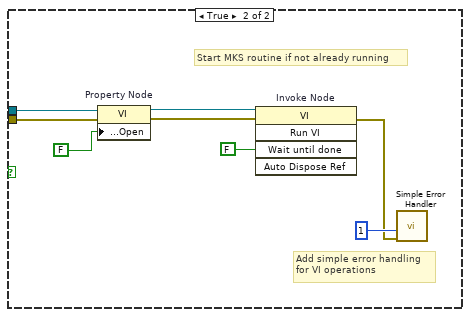
[diagram p5: hidden frame]
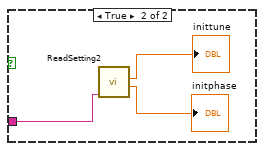
[diagram p6: hidden frame]
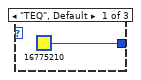
[diagram p8: hidden frame]
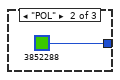
[diagram p9: hidden frame]
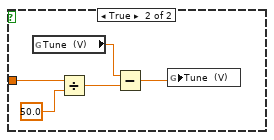
[diagram p10: hidden frame]
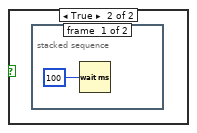
[diagram p11: hidden frame]
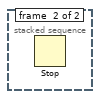
[diagram p12: hidden frame]
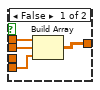
[diagram p13: hidden frame]
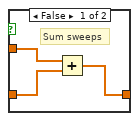
[diagram p14: hidden frame]
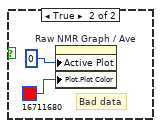
[diagram p15: hidden frame]
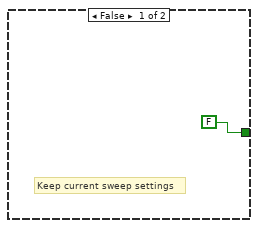
[diagram p17: hidden frame]
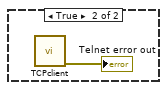
[diagram p18: hidden frame]
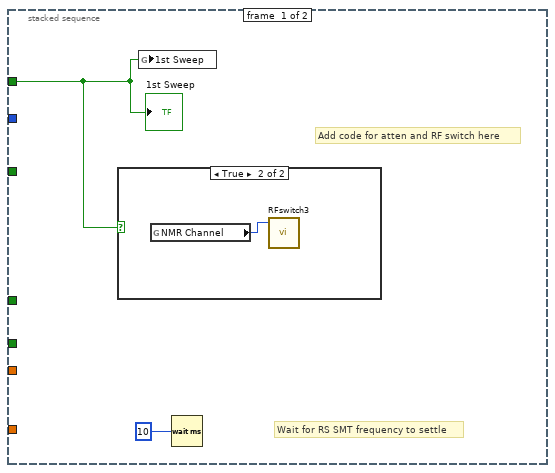
[diagram p19: hidden frame]
diagram:
  n1 = String To Path(string="C:\\users\\Ptgroup\\Desktop\\kleinjan\\MKS\\Task - Pressure & Flow.vi") -> (path=w8:path)
  n2 = Open VI Reference "Open VI Ref"(vi path=w8) -> (vi reference=w5:refnum<vi>, error out=w6:errorcluster)  [unwired: 5 in]
  n3 = String To Path(string="C:\\users\\Ptgroup\\Desktop\\rssmt\\Tune.vi") -> (path=w4:path)
  n4 = Open VI Reference "Open VI Ref"(vi path=w4) -> (vi reference=w2:refnum<vi>, error out=w1:errorcluster)  [unwired: 5 in]
  n5 = stacked-sequence {
    tunnel: w5 -> [w12 w77 w339]
    tunnel: w6 -> [w11 w76 w338]
    tunnel: w2 -> [_ w70 _]
    tunnel: w1 -> [_ w74 _]
    frame #0 {
      # "Prompt for text inputs"
      # "Load channel settings if needed"
      # "Open global planel"
      n6 = call "prompt.vi"("Enable"="Prompt?") -> ("Measurement"=w25:enum16{"TEQ", "POL", "QCV"}, "Run comment"=w24:string, "Q curve comment"=w23:string, "Q curve file"=w22:string, "TE Comment"=w21:string, "TE peak file"=w20:string)  [unwired: 11 in, 2 out]
      n7 = case shown="True" "Open Global Panel" {
        frame False {
        }
        frame True {
          n8 = vi-ref "Global 2.vi"() -> (w68:refnum<vi>)
          n9 = invoke class="VI" method="FP.Open"(reference=w68, "Activate"=TRUE, "State"=T1."Standard") -> ()  [unwired: 2 in, 5 out]
        }
      }
      n10 = feedback #1 "Feedback Node"() -> (w19:string)  [unwired: 1 in]
      n11 = feedback-in #1("NMR Channel Select") -> ()
      n12 = global write "Global 2.vi" "Tune file"("NMR Channel Select") -> ()
      n13 = global write "Global 2.vi" "Measurement"(w25) -> ()
      n14 = global write "Global 2.vi" "Q curve file"(w22) -> ()
      n15 = global write "Global 2.vi" "TEQ Comment"(w21) -> ()
      n16 = global write "Global 2.vi" "Q Comment"(w23) -> ()
      n17 = global write "Global 2.vi" "Commentary"(w24) -> ()
      n18 = global write "Global 2.vi" "TEQ file"(w20) -> ()
      n19 = Not Equal?(x=w19, y="NMR Channel Select") -> (x != y?=w18:bool)
      n20 = case shown="False" w18 {
        tunnel: "NMR Channel Select" -> [_ w65]
        frame False {
        }
        frame True {
          n21 = call "ReadSetting2.vi"("Data Filename"=w65) -> ("Phase"=→"initphase":dbl, "Tune"=→"inittune":dbl)  [unwired: 1 out]
        }
      }
      n22 = global read "Global 2.vi" "UsePython"() -> (w9:bool)
      n23 = case shown="False" w9 {
        frame False {
        }
        frame True {
          n24 = while {
            stop <- w28 stop-if-true
            n25 = flat-sequence {
              tunnel: [w45] -> w28
              frame #0 {
                w29 = TRUE  # run minimized?
                w30 = FALSE  # wait until completion?
                # "Start python analyzer in background"
                n26 = Wait (ms)(milliseconds to wait=100) -> ()  [unwired: 1 out]
                n27 = call <vilib>:"System Exec.vi"("run minimized? (F)"=w29, "wait until completion? (T)"=w30, "command line"="cmd /c taskkill /im python.exe /f") -> ()  [unwired: 5 in, 4 out]
              }
              frame #1 {
                n28 = Wait (ms)(milliseconds to wait=1000) -> ()  [unwired: 1 out]
              }
              frame #2 {
                w40 = FALSE  # run minimized?
                w41 = FALSE  # wait until completion?
                # "Start python analyzer in background"
                n29 = String To Path(string="C:\\Users\\plm\\Desktop\\NMRFastAna") -> (path=w35:path)
                n30 = call <vilib>:"System Exec.vi"("run minimized? (F)"=w40, "wait until completion? (T)"=w41, "working directory"=w35, "command line"="cmd /c python NMRFastAna.py --host=127.0.0.1 --port=10023 --qcvpath=c:\\Users\\plm\\Desktop\\rssmt\\data\\config") -> ("error out"=w36:errorcluster, "return code"=→"return code":i32, "standard error"=→"standard error":string, "standard output"=→"standard output":string)  [unwired: 4 in]
                n31 = call <vilib>:"Simple Error Handler.vi"("error in (no error)"=w36) -> ()  [unwired: 1 in, 8 out]
              }
              frame #3 {
                n32 = Wait (ms)(milliseconds to wait=100) -> ()  [unwired: 1 out]
              }
              frame #4 {
                n33 = case shown="False" FALSE {
                  tunnel: [TRUE w50] -> w45
                  frame False {
                  }
                  frame True {
                    n34 = call "TCPclientpython.vi"("Input Command"="test?") -> ("Telnet error"=w48:errorcluster, "Command and Results"=w53:string)  [unwired: 4 in, 1 out]
                    n35 = Unbundle By Name(w48) -> ("status"=w47:bool)
                    n36 = Equal?(x=w53, y="ok?") -> (x = y?=w51:bool)
                    n37 = Not(x=w47) -> (.not. x?=w49:bool)
                    n38 = And(x=w51, y=w49) -> (x .and. y?=w50:bool)
                  }
                }
                "Python OK" <- w45
              }
            }
          }
        }
      }
      n39 = property on="Property Node" class="VI"(reference=w12, error in=w11) -> (reference out=w14:refnum<vi>, error out=w13:errorcluster, "Exec.State"=w15:T2)
      n40 = Not Equal?(x=2, y=w15) -> ()  [unwired: 1 out]
      n41 = case shown="False" FALSE {
        tunnel: w14 -> [_ w59]
        tunnel: w13 -> [_ w58]
        frame False {
        }
        frame True {
          # "Start MKS routine if not already running"
          # "Add simple error handling\nfor VI operations"
          n42 = property on="Property Node" class="VI"(reference=w59, error in=w58, "Front Panel Window:Open"=FALSE ("Front Panel.Open")) -> (reference out=w57:refnum<vi>, error out=w56:errorcluster)
          n43 = invoke on="Invoke Node" class="VI" method="Run VI"(reference=w57, error in=w56, "Wait until done"=FALSE) -> (error out=w60:errorcluster)  [unwired: 2 in, 4 out]
          n44 = call <vilib>:"Simple Error Handler.vi"("type of dialog (OK msg:1)"=1, "error in (no error)"=w60) -> ()  [unwired: 3 in, 5 out]
        }
      }
    }
    frame #1 {
      w75 = dbl[] []
      # "Netburner"
      # "Improved mean"
      n45 = global read "Global 2.vi" "Measurement"() -> (w79:enum16{"TEQ", "POL", "QCV"})
      "Measurement" <- w79
      n46 = case shown="\"QCV\"" w79 {
        tunnel: [u32 16775210 ("Color Box 2") u32 3852288 ("Color Box 2") u32 16711680 ("Color Box 2")] -> w78
        frame "TEQ", Default {
        }
        frame "POL" {
        }
        frame "QCV" {
        }
      }
      "Color Box" <- w78
      n47 = global write "RunNumberGlobal.vi" "RunNumber"("RunNumber") -> ()
      n48 = property on="Property Node" class="VI"(reference=w70, error in=w74, "Front Panel Window:Open"="Tune?") -> ()  [unwired: 2 out]
      n49 = global read "Global 2.vi" "Center Freq (MHz)"() -> (w96:dbl)
      n50 = local read "initphase"() -> (w71:dbl)
      n51 = global read "Global 2.vi" "Step Width (MHz)"() -> (w94:dbl)
      n52 = local read "inittune"() -> (w72:dbl)
      n53 = global read "Global 2.vi" "# of Sweeps"() -> (w98:i32)
      n54 = global read "Global 2.vi" "Freq Span (MHz)"() -> (w95:dbl)
      n55 = global read "Global 2.vi" "RF Level (dBm)"() -> (w97:dbl)
      n56 = global read "Global 2.vi" "Quality cuts"() -> (w93:bool)
      n57 = global write "Global 2.vi" "IP Address"("VME IP Address") -> ()
      n58 = call "ReadQcurve.vi"() -> ("Array"=w84:dbl[])  [unwired: 2 in]
      n59 = Get Date/Time In Seconds() -> (seconds since 1Jan1904=w99:timestamp)
      n60 = To Double Precision Float(number=w99) -> (double precision float=w85:dbl)
      n61 = for {
        N: w98 -> [_]
        tunnel: [w248] -> w101 mode=indexing
        tunnel: w93 -> [w217]
        tunnel: w96 -> [w192]
        tunnel: w95 -> [w204]
        tunnel: w94 -> [w191]
        tunnel: "R&S GPIB Addr (28)" -> [w245]
        tunnel: w97 -> [w244]
        tunnel: w85 -> [w141]
        tunnel: w84 -> [w237]
        tunnel: [w207] -> w87
        tunnel: w77 -> [w171]
        tunnel: w76 -> [w170]
        shift-right: [w163] -> _
        shift-left: w75 -> [w162]
        shift-left: w75 -> [w153]
        shift-left: w75 -> [w161]
        shift-left: w75 -> [w160]
        shift-left: w75 -> [w159]
        shift-left: w75 -> [w158]
        shift-left: w75 -> [w157]
        shift-left: w75 -> [w156]
        shift-left: w75 -> [w155]
        shift-left: w75 -> [w154]
        tunnel: w72 -> [w145]
        tunnel: w71 -> [w144]
        i -> [w151]
        stop <- w143 stop-if-true
        (unwired) 1
        w197 = TRUE
        w212 = 4.9  # Vmax-0.1
        # "Amplify TEQ signal\nfor display"
        # "Adjust tune"
        # "Average signal or noise"
        # "Check voltage limits"
        # "Ave"
        # "Max Pedestal"
        # "Gain sel"
        # "F=real Q"
        # "Real Qcurve\nor quadratic"
        # "+-5V"
        # "Change data plot color if bad"
        # "Max IF offset (V)"
        # "Fmax"
        # "Fmax"
        # "Time"
        # "Vmin"
        # "Raw data"
        # "Corrected Data"
        # "Fcen"
        # "delta F"
        # "# steps"
        # "ADC range"
        # "sweep #"
        # "Set D/A converters, collect data, step frequency upwards, repeat until end of span"
        # "Calculates Q curve"
        # "Removes baseline drift"
        # "Bad voltage or pedestal?"
        # "# steps"
        # "Calculate Fstart"
        # "delta F step"
        n62 = Equal To 0?(x=w151) -> (x = 0?=w250:bool)
        n63 = Divide(x=w204, y=sgl 2.0) -> (x/y=w254:dbl)
        n64 = Subtract(x=w192, y=w254) -> (x-y=w195:dbl)
        n65 = local read "Tune?"() -> (w122:bool)
        n66 = call "Tune.vi"("Init Phase V"=w144, "Init Tune V"=w145, "Tune"=w122) -> ()  [unwired: 9 in]
        n67 = Multiply(x=500.0, y=w204) -> (x*y=w203:dbl)
        n68 = case shown="True" w250 {
          tunnel: w192 -> [_ w301]
          tunnel: w203 -> [_ w302]
          tunnel: [FALSE TRUE] -> w249
          tunnel: w245 -> [_ w298]
          tunnel: w244 -> [_ w297]
          frame False {
            # "Keep current sweep settings"
          }
          frame True {
            # "VME\nReset?"
            # "First sweep"
            # "SETUP RF LEVEL,  FREQUENCY SCAN\nand TURN RF ON. RESET VONTROLLER"
            n69 = case shown="False" FALSE {
              frame False {
              }
              frame True {
                n70 = call "TCPclient.vi"() -> ("Telnet error"=→"Telnet error out":errorcluster)  [unwired: 4 in, 3 out]
              }
            }
            n71 = call "NMRFMsweep.vi"("Center Freq (MHz)"=w301, "Freq Span (kHz)"=w302, "RF Level (dBm)"=w297, "Program"=TRUE, "GPIB Addr (28)"=w298) -> ("error out"=→"SMT error out":errorcluster)  [unwired: 2 in]
          }
        }
        n72 = Add(x=w195, y=w204) -> (x+y=w241:dbl)
        n73 = global read "Global 2.vi" "Subtract Q curve"() -> (w229:bool)
        n74 = global read "Global 2.vi" "Amp of Q curve"() -> (w230:dbl)
        n75 = Select(t=w230, s=w229, f=0.0) -> (s? t:f=w234:dbl)
        n76 = Multiply(x=w237, y=w234) -> (x*y=w236:dbl[])
        n77 = Divide(x=w204, y=w191) -> (x/y=w256:dbl)
        n78 = global read "Global 2.vi" "Invert Polarity"() -> (w179:bool)
        n79 = global read "Global 2.vi" "Gain"() -> (w183:enum16{"LOW", "HI", "MAX"})
        n80 = global read "Global 2.vi" "IFoffset (V)"() -> (w206:dbl)
        n81 = global read "Global 2.vi" "Tune  (V)"() -> (w231:dbl)
        n82 = To Word Integer(number=w256) -> (16bit integer=w253:i16)
        n83 = To Double Precision Float(number=w183) -> (double precision float=w182:dbl)
        n84 = call "Gainsel.vi"("Gain"=w183) -> ("LO"=w209:bool, "MAX"=w208:bool)  [unwired: 1 out]
        n85 = Increment(x=w253) -> (x+1=w152:i16)
        n86 = for {
          N: w152 -> [_]
          tunnel: w162 -> [w266] mode=indexing
          tunnel: w161 -> [w274] mode=indexing
          tunnel: w160 -> [w273] mode=indexing
          tunnel: w159 -> [w272] mode=indexing
          tunnel: w158 -> [w271] mode=indexing
          tunnel: w157 -> [w270] mode=indexing
          tunnel: w156 -> [w269] mode=indexing
          tunnel: w155 -> [w268] mode=indexing
          tunnel: w154 -> [w267] mode=indexing
          tunnel: w153 -> [w275] mode=indexing
          tunnel: [w263] -> w150 mode=indexing
          # "Running sum of 10 sweeps"
          n87 = Compound Arithmetic op=ADD(w266, w275, w274, w273, w272, w271, w270, w269, w268, w267) -> (w264:dbl)
          n88 = Divide(x=w264, y=10) -> (x/y=w263:dbl)
        }
        n89 = Boolean To (0,1)(Boolean=w179) -> (0, 1=w180:i16)
        n90 = Increment(x=w151) -> (x+1=w215:i32)
        "Sweep #" <- w215
        n91 = To Double Precision Float(number=w152) -> (double precision float=w190:dbl)
        n92 = To Double Precision Float(number=w180) -> (double precision float=w178:dbl)
        n93 = stacked-sequence {
          tunnel: [_ w324] -> w193
          tunnel: [_ w328] -> w105
          tunnel: w152 -> [_ w322]
          tunnel: w206 -> [_ w319]
          tunnel: w209 -> [_ w326]
          tunnel: w249 -> [w304 _]
          tunnel: w231 -> [_ w320]
          tunnel: [_ w313] -> w188
          tunnel: [_ w312] -> w135
          tunnel: [_ w320] -> w187
          tunnel: [_ w319] -> w186
          tunnel: [_ w318] -> _
          tunnel: w208 -> [_ w318]
          tunnel: [_ w311] -> w181
          tunnel: w179 -> [_ w310]
          tunnel: [_ w307] -> w177
          frame #0 {
            # "Add code for atten and RF switch here"
            # "Wait for RS SMT frequency to settle"
            n94 = case shown="True" w304 {
              frame False {
              }
              frame True {
                n95 = global read "Global 2.vi" "NMR Channel"() -> (w306:i32)
                n96 = call "RFswitch3.vi"("RF Channel"=w306) -> ()  [unwired: 4 in, 1 out]
              }
            }
            n97 = global write "Global 2.vi" "1st Sweep"(w304) -> ()
            n98 = Wait (ms)(milliseconds to wait=10) -> ()  [unwired: 1 out]
            "1st Sweep" <- w304
          }
          frame #1 {
            # "+3.3V"
            # "Offset"
            # "Tune"
            # "Stand dev."
            # "ADCval"
            # "ACQUIRE SINGLE CHANNEL DATA\nCALCULATE MEAN AND ERROR\nSETUP FOR NEG IF VOLTAGE"
            # "# of freq steps"
            n99 = global read "Global 2.vi" "IF / LOG Det"() -> (w309:bool)
            n100 = Boolean To (0,1)(Boolean=w309) -> (0, 1=w308:i16)
            n101 = case shown="True" w309 {
              tunnel: w326 -> [w333 w334]
              tunnel: [w330 w335] -> w323
              frame False {
                n102 = Select "ADC Chan"(t=1, s=w333, f=0) -> (s? t:f=w330:i32)
              }
              frame True {
                n103 = Select "ADC Chan"(t=2, s=w334, f=3) -> (s? t:f=w335:i32)
              }
            }
            n104 = To Double Precision Float(number=w308) -> (double precision float=w307:dbl)
            n105 = global read "Global 2.vi" "# Sample/step"() -> (w315:i32)
            n106 = global read "Global 2.vi" "Tank RF"() -> (w316:bool)
            n107 = global read "Global 2.vi" "IF Atten (dB)"() -> (w314:i8)
            n108 = global read "Global 2.vi" "Logoffset (V)"() -> (w317:dbl)
            n109 = Not(x=w316) -> (.not. x?=w321:bool)
            n110 = global read "Global 2.vi" "Phase (V)"() -> (w311:dbl)
            n111 = call "Netburner_cntlTCP.vi"("Phase Volt"=w311, "Tune Volt"=w320, "# Data"=w315, "IF Atten (dB)"=w314, "NMR ADC"=w323, "Hi Gain"=w318, "Tank RF"=w321, "LogOff Volt"=w317, "IFOff Volt"=w319, "# f steps"=w322) -> ("Temp (C)"=w313:dbl, "ADC value"=w325:dbl[], "ADC Std Dev"=w324:dbl, "Volts"=w312:dbl)  [unwired: 2 out]
            "Temp (C)" <- w313
            "+3.3V supply" <- w312
            n112 = global write "Global 2.vi" "+3V supply"(w312) -> ()
            n113 = global write "Global 2.vi" "Temp (C)"(w313) -> ()
            n114 = Negate(x=w325) -> (-x=w327:dbl[])
            n115 = Wait (ms)(milliseconds to wait=1) -> ()  [unwired: 1 out]
            n116 = Select(t=w327, s=w310, f=w325) -> (s? t:f=w328:dbl[])
          }
        }
        n117 = global write "Global 2.vi" "Sweep #"(w215) -> ()
        n118 = call "Qcorrect.vi"("Subtract Q curve"=w229, "Nstep"=w152, "Max Gain"=w208, "Amp of Q curve"=w230, "Step Width (MHz)"=w191, "Center Freq (MHz)"=w192) -> ("Start"=w251:i32, "Array"=w252:dbl[])
        n119 = global read "Global 2.vi" "Real/Quad Q curve"() -> (w228:bool)
        n120 = To Double Precision Float(number=w215) -> (double precision float=w189:dbl)
        n121 = Array Subset "Array Subset"(array=w252, index=w251, length=w152) -> (w238:dbl[])
        n122 = property on="Property Node" class="VI"(reference=w171, error in=w170) -> ("Exec.State"=w173:T2)  [unwired: 2 out]
        n123 = global read "Global 2.vi" "AutoTune"() -> (w226:bool)
        n124 = Select(t=w238, s=w228, f=w236) -> (s? t:f=w165:dbl[])
        n125 = Not(x=w226) -> (.not. x?=w239:bool)
        n126 = Equal?(x=2, y=w173) -> (x = y?=→"He readback":bool)
        n127 = Not(x="Stop Run") -> (.not. x?=w143:bool)
        n128 = Greater?(x=w206, y=7.5) -> (0:w242:bool)
        n129 = Not(x=w242) -> (.not. x?=w222:bool)
        "RF level OK" <- w222
        n130 = global write "Global 2.vi" "RF OK"(w222) -> ()
        n131 = case shown="False" w143 {
          frame False {
          }
          frame True {
            n132 = stacked-sequence {
              frame #0 {
                n133 = Wait (ms)(milliseconds to wait=100) -> ()  [unwired: 1 out]
              }
              frame #1 {
                n134 = Stop() -> ()  [unwired: 1 in]
              }
            }
          }
        }
        n135 = global read "Global 2.vi" "Amp of Q curve"() -> (w184:dbl)
        n136 = To Double Precision Float(number=w215) -> (double precision float=w210:dbl)
        n137 = global read "Global 2.vi" "RemovePed"() -> (w227:bool)
        n138 = Equal To 0?(x=w151) -> (x = 0?=w214:bool)
        n139 = call "RemoveQandP.vi"("Subtract Ped?"=w227, "Qcurve"=w165, "Raw data"=w105) -> ("Ped L-R"=w116:dbl, "Corrected data"=w200:dbl[], "Ped Offfset"=w123:dbl)
        "Pedestal (V)" <- w123
        n140 = Multiply(x=w123, y=10.0) -> (x*y=w232:dbl)
        n141 = call "Autozero.vi"("Vmin (V)"=w232, "IFoffset (V)"=w206, "Enable"=w239, "Max Gain"=w208) -> ()
        n142 = global write "Global 2.vi" "Pedestal Offset"(w123) -> ()
        n143 = global read "Global 2.vi" "Gauss Fit"() -> (w225:bool)
        n144 = global write "Global 2.vi" "Sample RMS (V)"(w193) -> ()
        n145 = Get Date/Time In Seconds() -> (seconds since 1Jan1904=w149:timestamp)
        n146 = Subtract(x=w135, y=3.3) -> (x-y=w137:dbl)
        n147 = global write "Global 2.vi" "Temperature (C)"(w188) -> ()
        n148 = Array Max & Min "Array Max"(array=w200) -> (max value=w185:dbl)  [unwired: 3 out]
        n149 = Absolute Value(x=w137) -> (abs(x)=w136:dbl)
        n150 = call-poly <vilib>:"Power Spectrum.vi"("X"=w105) -> ("Power Spectrum"=w205:dbl[])  [unwired: 1 out]
        n151 = Less?(x=w136, y=0.1) -> (x < y?=→"+3.3V OK":bool)
        n152 = global read "Global 2.vi" "Calib Constant"() -> (w140:dbl)
        n153 = Absolute Value ("Abs Value")(x=w116) -> (abs(x)=w246:dbl)
        n154 = Negate(x=w116) -> (-x=w121:dbl)
        "Pedestal Diff (V)" <- w121
        n155 = call "FitData.vi"("Fit?"=w225, "Fmax"=w241, "Fmin"=w195, "Yarray"=w200) -> ("Peak Area (mV-MHz)"=w107:dbl, "Center Freq (MHz)"=w110:dbl, "NMR Graph + Fit"=w221:cluster{cluster{dbl, "Numeric":dbl}[]}[])  [unwired: 2 out]
        n156 = Build Array (concatenate) "Header + Data"(w192, w191, w190, w189, w188, w135, w187, w186, w181, w107, w184, w140, w182, w178, w177, w105) -> (w142:dbl[])
        n157 = global write "Global 2.vi" "NMR Graph + Fit"(w221) -> ()
        n158 = Square Root(x=w205) -> (sqrt(x)=w201:dbl[])
        "FFT Vrms" <- w201
        n159 = global read "Global 2.vi" "Subtract Q curve"() -> (w112:bool)
        n160 = call "SaveTune.vi"("Array"=w142, "Save Data to File"="Save Tune", "Ext time (sec)"=w141, "RawSignal"=w105) -> ()
        n161 = global write "Global 2.vi" "Pedestal Difference"(w121) -> ()
        n162 = global write "Global 2.vi" "Pedestal Diff (V)"(w121) -> ()
        n163 = Select(t=w105, s=w197, f=w201) -> (s? t:f=w163:dbl[])
        n164 = Format Date/Time String(time format string (%c)="%c", seconds (now)=w149) -> (date/time string=→"Date / Time":string)  [unwired: 1 in]
        n165 = call "SaveData.vi"("Quad sub area"=w107, "Ext time (sec)"=w141, "Array"=w142) -> ("Frequency"=w111:dbl, "Area"=w139:dbl, "ADC value"=w131:dbl[])  [unwired: 1 out]
        n166 = feedback #2 "Feedback Node"() -> (w213:dbl[])  [unwired: 1 in]
        n167 = case shown="True" w214 {
          tunnel: w163 -> [w285 w287]
          tunnel: [w284 w287] -> w211
          tunnel: w213 -> [w286 _]
          frame False {
            # "Sum sweeps"
            n168 = Add(x=w286, y=w285) -> (x+y=w284:dbl[])
          }
          frame True {
            # "Initialize"
          }
        }
        n169 = feedback-in #2(w211) -> ()
        n170 = Divide(x=w211, y=w210) -> (x/y=w164:dbl[])
        n171 = Multiply(x=w140, y=w185) -> (x*y=w106:dbl)
        "Peak amp (mV)" <- w106
        "Peak Amp" <- w106
        n172 = Select(t=0.1, s=w208, f=0.1) -> (s? t:f=w216:dbl)
        n173 = Multiply(x=w139, y=w140) -> (x*y=w115:dbl)
        n174 = Multiply(x=w107, y=w140) -> (x*y=w113:dbl)
        n175 = Not(x=w112) -> (.not. x?=w109:bool)
        n176 = Greater?(x=w246, y=w216) -> (0:w218:bool)
        n177 = call "ADCok.vi"("PedOK"=w218, "Array"=w105, "Vmax-1/2"=w212) -> ("ADC voltages OK"=w224:bool, "Allok"=w240:bool)  [unwired: 1 out]
        "ADC volts OK" <- w224
        n178 = global read "Global - Pressure & Flow.vi" "Task3 Temperature"() -> (→"He temp (K)":dbl)
        n179 = global read "Global - Pressure & Flow.vi" "Task3 Pressure"() -> (→"He press (torr)":dbl)
        n180 = And(x=w240, y=w217) -> (x .and. y?=w247:bool)
        n181 = case shown="False" w240 {
          frame False {
            # "All OK"
            n182 = property on="Raw NMR Graph / Ave" class="WFGraph (strict)"("Active Plot"=0, "Plot.Plot Color"=u32 13145856) -> ()  [unwired: 2 in, 2 out]
          }
          frame True {
            # "Bad data"
            n183 = property on="Raw NMR Graph / Ave" class="WFGraph (strict)"("Active Plot"=0, "Plot.Plot Color"=u32 16711680) -> ()  [unwired: 2 in, 2 out]
          }
        }
        n184 = Not(x=w218) -> (.not. x?=w223:bool)
        "Pedestal volts OK" <- w223
        n185 = Select(t=w115, s=w109, f=w113) -> (s? t:f=w114:dbl)
        "Polarization %" <- w114
        "Polarization" <- w114
        n186 = global read "Global 2.vi" "Subtract Q curve"() -> (w166:bool)
        n187 = Select(t=w195, s=w197, f=0.0) -> (s? t:f=w194:dbl)
        n188 = Select(t=w191, s=w197, f=1.0) -> (s? t:f=w198:dbl)
        n189 = global write "Global 2.vi" "Pedestal OK"(w223) -> ()
        n190 = Select(t=w111, s=w109, f=w110) -> (s? t:f=w108:dbl)
        "Peak center (MHz)" <- w108
        n191 = global write "Global 2.vi" "ADC volts OK"(w224) -> ()
        n192 = case shown="True" w247 {
          tunnel: [w292 -99.0] -> w248
          tunnel: w114 -> [w292 _]
          frame False {
            # "Data OK"
          }
          frame True {
            # "flag it bad"
          }
        }
        n193 = global write "Global 2.vi" "Peak center (MHz)"(w108) -> ()
        n194 = global write "Global 2.vi" "Peak Height"(w114) -> ()
        n195 = global read "Global 2.vi" "AutoFreq"() -> (w117:bool)
        n196 = local read "Tune?"() -> (w120:bool)
        n197 = global write "Global 2.vi" "Peak amp (V)"(w106) -> ()
        n198 = global read "Global 2.vi" "Measurement"() -> (w129:enum16{"TEQ", "POL", "QCV"})
        n199 = global write "Global 2.vi" "Peak area (mV-MHz)"(w114) -> ()
        n200 = Not(x=w120) -> (.not. x?=w118:bool)
        n201 = And(x=w117, y=w118) -> (x .and. y?=w119:bool)
        n202 = Not Equal?(x=w129, y=1) -> (x != y?=w127:bool)
        n203 = case shown="False" w119 {
          tunnel: w116 -> [_ w257]
          frame False {
          }
          frame True {
            n204 = global read "Global 2.vi" "Tune  (V)"() -> (w259:dbl)
            n205 = Divide(x=w257, y=50.0) -> (x/y=w260:dbl)
            n206 = Subtract(x=w259, y=w260) -> (x-y=w258:dbl)
            n207 = global write "Global 2.vi" "Tune  (V)"(w258) -> ()
          }
        }
        n208 = Select(t=10.0, s=w127, f=1.0) -> (s? t:f=w124:dbl)
        n209 = Multiply(x=w131, y=w124) -> (x*y=w130:dbl[])
        n210 = case shown="True" w166 {
          tunnel: w163 -> [w279 w283]
          tunnel: [w278 w282] -> w167
          tunnel: w165 -> [_ w281]
          tunnel: w150 -> [w277 w280]
          tunnel: w130 -> [w276 _]
          frame False {
            n211 = Build Array(w279, w277, w276) -> (w278:dbl[][])
          }
          frame True {
            n212 = Build Array(w283, w280, w281) -> (w282:dbl[][])
          }
        }
        n213 = Bundle(w194, "Step Width (MHz)"=w198, w167) -> (→"Raw NMR Graph / Ave":cluster{dbl, "Step Width (MHz)":dbl, dbl[][]})  [unwired: 1 in]
        n214 = global read "Global 2.vi" "Fit OK"() -> (→"Qsub OK":bool)
        n215 = Build Array (concatenate) "Build Array"(w194, w198, w164) -> (w207:dbl[])
      }
      n216 = call "DataQA.vi"("Quality cuts"=w93, "Data In"=w101) -> ("Data Out"=w100:dbl[])
      n217 = global read "Global 2.vi" "Save Data to File"() -> (w86:bool)
      n218 = call <vilib>:"Std Deviation and Variance.vi"("X"=w100) -> ("mean"=w91:dbl, "standard deviation"=w81:dbl)  [unwired: 1 in, 1 out]
      "Polarization %" <- w91
      n219 = Multiply(x=w81, y=1.0) -> (x*y=→"Pol sdev":dbl)
      n220 = call "PeakHisto.vi"("Data Out"=w100) -> ("XY Graph"=w89:cluster{"Y":dbl[], "Y":dbl[]}[])
      "Peak Height Distribution" <- w89
      n221 = global write "Global 2.vi" "Peak Height Distribution"(w89) -> ()
      n222 = global write "Global 2.vi" "Peak mean (V)"(w91) -> ()
      n223 = call "SaveDataAve.vi"("Array"=w87, "Save Data to File"=w86) -> ()  [unwired: 1 in, 1 out]
      n224 = Array Size(array=w100) -> (size(s)=w90:i32)
      "# Good Spectra" <- w90
      n225 = global write "Global 2.vi" "# Good Spectra"(w90) -> ()
      n226 = Divide(x=w91, y=w81) -> (x/y=w92:dbl)
      "S/N" <- w92
      n227 = global write "Global 2.vi" "S/N"(w92) -> ()
    }
    frame #2 {
      n228 = property on="Property Node" class="VI"(reference=w339, error in=w338) -> (reference out=w341:refnum<vi>, error out=w340:errorcluster, "Exec.State"=w343:T2)
      n229 = Equal?(x=2, y=w343) -> (x = y?=w342:bool)
      n230 = case shown="True" w342 {
        tunnel: w341 -> [_ w350]
        tunnel: w340 -> [_ w349]
        frame False {
        }
        frame True {
          # "Stop MKS routine and close panel if running"
          # "Add simple error handling\nfor VI operations"
          n231 = invoke on="Invoke Node" class="VI" method="Abort VI"(reference=w350, error in=w349) -> (reference out=w347:refnum<vi>, error out=w346:errorcluster)  [unwired: 1 in, 1 out]
          n232 = property on="Property Node" class="VI"(reference=w347, error in=w346, "Front Panel Window:Open"=FALSE) -> (error out=w345:errorcluster)  [unwired: 1 out]
          n233 = call <vilib>:"Simple Error Handler.vi"("type of dialog (OK msg:1)"=1, "error in (no error)"=w345) -> ()  [unwired: 3 in, 5 out]
        }
      }
    }
  }
